vi "UtilityLib.CSV write.vi"(1 "file (use dialog)":path, 2 "CSVArray":string[][](array[string]), 5 "error in":errorcluster) -> (19 "error out":errorcluster)   [LabVIEW 2014, in "UtilityLib.lvlib"]
doc: "Converts information from a 2-dim array and writes the array to a CSV file. The fields in the CSV file may be embedded in double quotes (\") . However, the information embedded in double quotes may not contain special characters like double quotes, carriage returns or line feeds."
uses:
  UtilityLib.lvlib
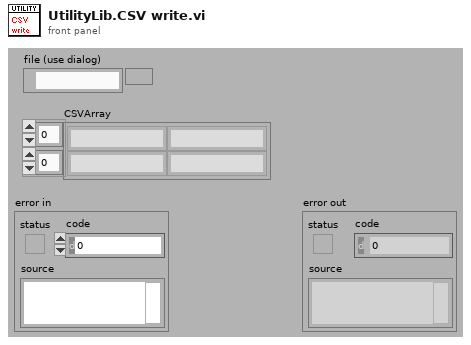
[diagram p1: front panel]
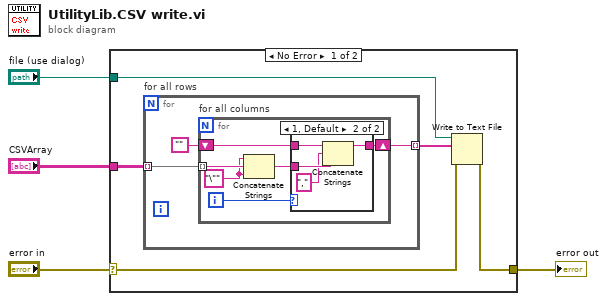
[diagram p0: block diagram]
diagram:
  n1 = case shown="No Error" "error in" {
    selector: "error in" -> [w6 w24]
    tunnel: [w5 w24] -> w4
    tunnel: "file (use dialog)" -> [w7 _]
    tunnel: "CSVArray" -> [w9 _]
    frame No Error {
      n2 = for "for all rows" {
        tunnel: w9 -> [w12] mode=indexing
        tunnel: [w10] -> w8 mode=indexing
        n3 = for "for all columns" {
          tunnel: w12 -> [w18] mode=indexing
          shift-right: [w14] -> w10
          shift-left: "" ("Empty String Constant") -> [w15]
          i -> [w16]
          w17 = "\"" ("string")
          n4 = Concatenate Strings(w17, w18, w17) -> (w13:string)
          n5 = case shown="1, Default" w16 {
            tunnel: w15 -> [_ w23]
            tunnel: [w19 w22] -> w14
            tunnel: w13 -> [w19 w21]
            frame 0 {
            }
            frame 1, Default {
              n6 = Concatenate Strings(w23, "," ("string"), w21) -> (w22:string)
            }
          }
        }
      }
      n7 = Write to Text File(file (use dialog)=w7, text=w8, error in=w6) -> (error out=w5:errorcluster)  [unwired: 1 in, 2 out]
    }
    frame Error {
    }
  }
  "error out" <- w4
